vi "set active handles.vi"(6 "serial numbers":string[](array[string]), 8 "error in (no error)":errorcluster, 9 "All Camera":T1[](array[typedef]), 10 "All Handles":variant[](array[variant]), 11 "Camera in":refnum<class "Camera.lvclass">) -> (0 "error out":errorcluster, 1 "Selected cameras":T1[](array[typedef]), 2 "Selected Handles":variant[](array[variant]), 3 "Camera out":refnum<class "Camera.lvclass">)   [LabVIEW 2022 SP3, in "Camera.lvlib" / "Camera.lvclass"]
uses:
  Camera.lvclass
  Resources/Type Defs/Physical Camera Assignment.ctl
  Camera.lvclass/Camera.ctl
  Resources/GLOBAL/GLOBAL Time-critical.vi
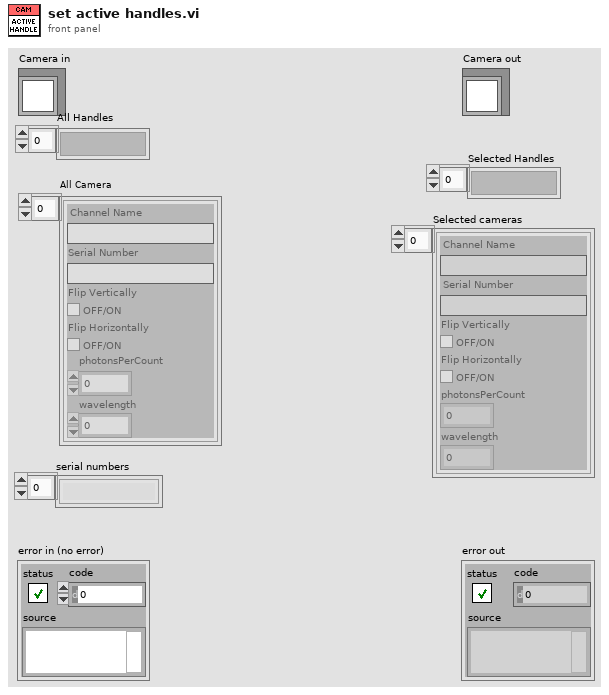
[diagram p1: front panel]
types:
  T1 = typedef "Physical Camera Assignment.ctl" = cluster{"Channel Name":string, "Serial Number":string, "Flip Vertically":bool, "Flip Horizontally":bool, "photonsPerCount":dbl, "wavelength":i16}
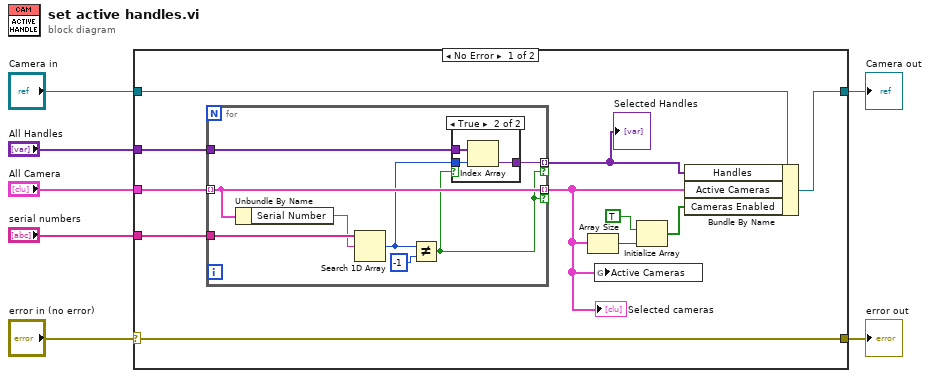
[diagram p0: block diagram]
diagram:
  n1 = case shown="No Error" "error in (no error)" {
    selector: "error in (no error)" -> [w18 w31]
    tunnel: [w18 w31] -> w6
    tunnel: [w16 w30] -> w4
    tunnel: "Camera in" -> [w17 w30]
    tunnel: "All Camera" -> [w12 _]
    tunnel: "serial numbers" -> [w11 _]
    tunnel: "All Handles" -> [w8 _]
    frame No Error {
      n2 = for {
        tunnel: w12 -> [w24] mode=indexing
        tunnel: w11 -> [w26]
        tunnel: [w24] -> w10 mode=indexing if=w20
        tunnel: [w22] -> w9 mode=indexing if=w20
        tunnel: w8 -> [w19]
        n3 = Unbundle By Name(w24) -> ("Serial Number"=w25:string)
        n4 = Search 1D Array(1D array=w26, element=w25) -> (index of element=w21:i32)  [unwired: 1 in]
        n5 = Not Equal?(x=w21, y=-1) -> (x != y?=w20:bool)
        n6 = case shown="True" w20 {
          tunnel: [_ w27] -> w22
          tunnel: w21 -> [_ w29]
          tunnel: w19 -> [_ w28]
          frame False {
          }
          frame True {
            n7 = Index Array(array=w28, index=w29) -> (element=w27:variant)
          }
        }
      }
      "Selected Handles" <- w9
      "Selected cameras" <- w10
      n8 = Array Size(array=w10) -> (size(s)=w15:i32)
      n9 = global write "GLOBAL Time-critical.vi" "Active Cameras"(w10) -> ()
      n10 = Initialize Array(TRUE, w15) -> (w13:bool[])
      n11 = Bundle By Name(cluster=w17, "Handles"=w9, "Active Cameras"=w10, "Cameras Enabled"=w13) -> (w16:refnum<class "Camera.lvclass">)
    }
    frame Error {
    }
  }
  "error out" <- w6
  "Camera out" <- w4
